vi "WPI_EncoderCache.vi"(8 "error in (no error)":errorcluster, 9 "EncoderToRelease":T1, 11 "Operation":T2) -> (0 "error out":errorcluster, 2 "EncoderAllocated":T1, 3 "Allocated":bool)   [LabVIEW 2017]
doc: "This software is licensed. Open the labview\\readme\\WPI Robotics Library Open Source License.txt file for more information."
uses:
  <vilib>/Rock Robotics/WPI/Encoder/WPI_EncoderCacheOp.ctl
  <vilib>/Rock Robotics/SystemInterfaces/Encoder/FPGA_EncoderIdx.ctl
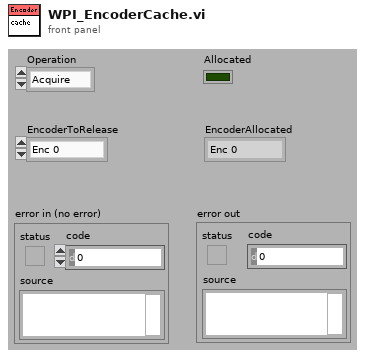
[diagram p1: front panel]
types:
  T1 = typedef "FPGA_EncoderIdx.ctl" = enum8{"Enc 0", "Enc 1", "Enc 2", "Enc 3", "Enc 4", "Enc 5", "Enc 6", "Enc 7", "Invalid"}
  T2 = typedef "WPI_EncoderCacheOp.ctl" = enum16{"Acquire", "Release"}
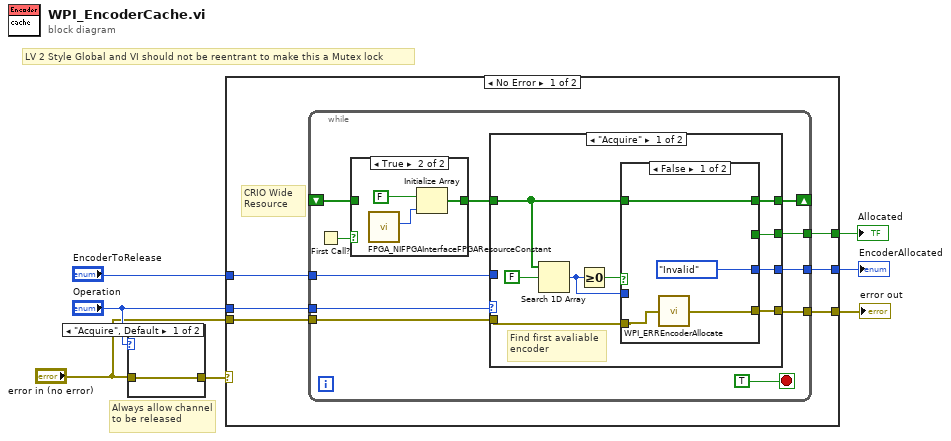
[diagram p0: block diagram]
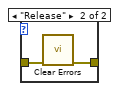
[diagram p2: hidden frame]
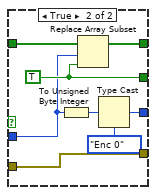
[diagram p3: hidden frame]
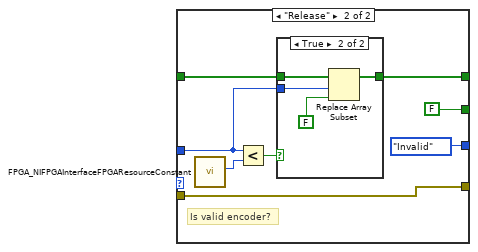
[diagram p4: hidden frame]
diagram:
  # "LV 2 Style Global and VI should not be reentrant to make this a Mutex lock"
  # "Always allow channel to be released"
  n1 = case shown="\"Acquire\", Default" "Operation" {
    tunnel: "error in (no error)" -> [w8 w10]
    tunnel: [w8 w9] -> w5
    frame "Acquire", Default {
    }
    frame "Release" {
      n2 = call <vilib>:"Clear Errors.vi"("error in (no error)"=w10) -> ("error out"=w9:errorcluster)  [unwired: 1 in, 5 out]
    }
  }
  n3 = case shown="No Error" w5 {
    selector: w5 -> [_ w66]
    tunnel: "Operation" -> [w16 _]
    tunnel: [w15 w66] -> w1
    tunnel: [w14 _] -> w7
    tunnel: "EncoderToRelease" -> [w12 _]
    tunnel: [w13 _] -> w4
    tunnel: "error in (no error)" -> [w11 _]
    frame No Error {
      # "CRIO Wide \nResource"
      n4 = while {
        shift-right: [w24] -> _
        shift-left: _ -> [w26]
        tunnel: w16 -> [w25]
        tunnel: w12 -> [w20]
        tunnel: [w23] -> w15
        tunnel: [w22] -> w14
        tunnel: [w19] -> w13
        tunnel: w11 -> [w17]
        stop <- TRUE stop-if-true
        n5 = First Call?() -> (First Call?: T/F=w27:bool)
        n6 = case shown="True" w27 {
          tunnel: w26 -> [w62 _]
          tunnel: [w62 w64] -> w21
          frame False {
          }
          frame True {
            n7 = call <vilib>:"FPGA_NIFPGAInterfaceFPGAResourceConstant.vi"() -> ("NumberOfEncoders"=w63:u32)  [unwired: 11 out]
            n8 = Initialize Array(FALSE, w63) -> (w64:bool[])
          }
        }
        n9 = case shown="\"Acquire\"" w25 {
          tunnel: w21 -> [w31 w56]
          tunnel: [w36 w55] -> w24
          tunnel: w20 -> [_ w51]
          tunnel: [w35 w49] -> w23
          tunnel: [w34 FALSE ("new element/subarray")] -> w22
          tunnel: [w33 FPGA_EncoderIdx."Invalid" ("EncoderToRelease")] -> w19
          tunnel: w17 -> [w28 w49]
          frame "Acquire" {
            # "Find first avaliable\nencoder"
            n10 = Search 1D Array(1D array=w31, element=FALSE) -> (index of element=w29:i32)  [unwired: 1 out]
            n11 = Greater Or Equal To 0?(x=w29) -> (x >= 0?=w30:bool)
            n12 = case shown="False" w30 {
              tunnel: w31 -> [w40 w47]
              tunnel: [w40 w46] -> w36
              tunnel: w29 -> [_ w42]
              tunnel: [w38 w41] -> w35
              tunnel: [_ w48] -> w34
              tunnel: [FPGA_EncoderIdx."Invalid" ("EncoderToRelease") w44] -> w33
              tunnel: w28 -> [w37 w41]
              frame False {
                n13 = call <vilib>:"WPI_ERREncoderAllocate.vi"("error in (no error)"=w37) -> ("ERRCounterAllocation"=w38:errorcluster)
              }
              frame True {
                w48 = TRUE ("new element/subarray")
                n14 = To Unsigned Byte Integer(number=w42) -> (unsigned 8bit integer=w43:u8)
                n15 = Replace Array Subset(array=w47, new element=w48, index=w42) -> (w46:bool[])
                n16 = Type Cast(type=FPGA_EncoderIdx."Enc 0" ("EncoderToRelease"), x=w43) -> (*(type *) &x=w44:T1)
              }
            }
          }
          frame "Release" {
            # "Is valid encoder?"
            n17 = call <vilib>:"FPGA_NIFPGAInterfaceFPGAResourceConstant.vi"() -> ("NumberOfEncoders"=w50:u32)  [unwired: 11 out]
            n18 = Less?(x=w51, y=w50) -> (x < y?=w52:bool)
            n19 = case shown="True" w52 {
              tunnel: w56 -> [w57 w61]
              tunnel: [w57 w60] -> w55
              tunnel: w51 -> [_ w58]
              frame False {
              }
              frame True {
                n20 = Replace Array Subset(array=w61, new element=FALSE ("new element/subarray"), index=w58) -> (w60:bool[])
              }
            }
          }
        }
      }
    }
    frame Error {
    }
  }
  "Allocated" <- w7
  "error out" <- w1
  "EncoderAllocated" <- w4
